vi "Auto-Cycle.vi"(8 "error in (no error)":errorcluster, 11 "SimAsync in":refnum<class "SimAsync.lvclass">) -> (0 "error out":errorcluster, 3 "SimAsync out":refnum<class "SimAsync.lvclass">)   [LabVIEW 2014, in "SimAsync.lvlib" / "SimAsync.lvclass"]
uses:
  SimAsync.lvclass
  DriverMasterAsync/builds/DriverMasterAsync.lvlibp/Modules/HAL/DriverMasterAsync/DriverMasterAsyncClass/DriverMasterAsync.lvclass
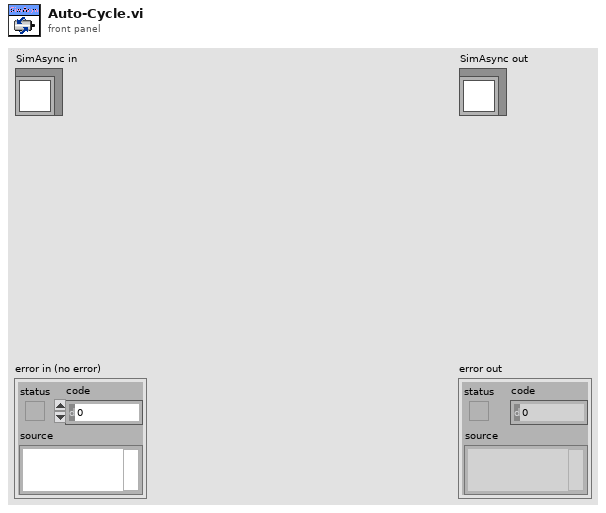
[diagram p1: front panel]
types:
  T1 = typedef "DriverMasterAsync.lvlibp/WINFAS 2 Data Queue.lvlib/Async Acquisition Data Cluster.ctl" = cluster{"Data":sgl[]}
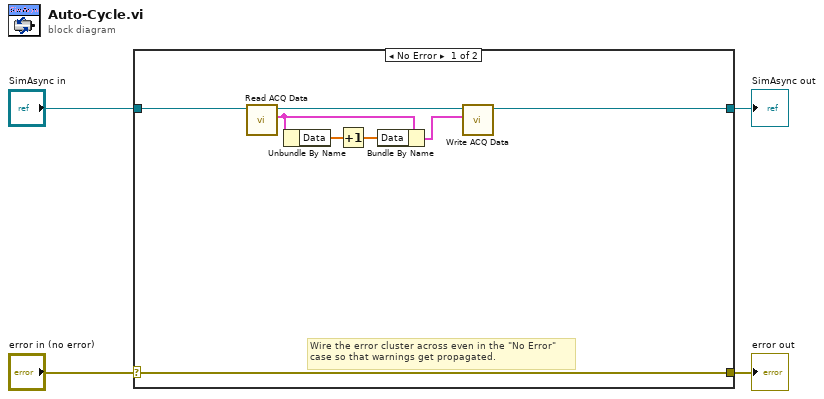
[diagram p0: block diagram]
diagram:
  n1 = case shown="No Error" "error in (no error)" {
    selector: "error in (no error)" -> [w12 w14]
    tunnel: [w12 w14] -> w3
    tunnel: [w5 w13] -> w1
    tunnel: "SimAsync in" -> [w6 w13]
    frame No Error {
      # "Wire the error cluster across even in the \"No Error\"\ncase so that warnings get propagated."
      n2 = call "Read ACQ Data.vi"("DriverMasterAsync in"=w6) -> ("ACQ Data"=w10:T1, "DriverMasterAsync out"=w11:refnum<class "SimAsync.lvclass">)  [unwired: 8 in, 1 out]
      n3 = Unbundle By Name(w10) -> ("Data"=w8:sgl[])
      n4 = Increment(x=w8) -> (x+1=w7:sgl[])
      n5 = Bundle By Name(cluster=w10, "Data"=w7) -> (w9:T1)
      n6 = call "Write ACQ Data.vi"("ACQ Data"=w9, "DriverMasterAsync in"=w11) -> ("DriverMasterAsync out"=w5:refnum<class "SimAsync.lvclass">)  [unwired: 8 in, 1 out]
    }
    frame Error {
    }
  }
  "error out" <- w3
  "SimAsync out" <- w1
